vi "snapAndEnqueueTester.vi"(11 "Session In":T2) -> ()   [LabVIEW 2013]
uses:
  <vilib>/userdefined/High Color/IMAQdx.ctl
  <vilib>/vision/driver/NI_Vision_Acquisition_Software.lvlib
  <resource>/objmgr/imaqdx.rc
panel:
  in  "stop":bool
  out "Image":T1(plugin-control)
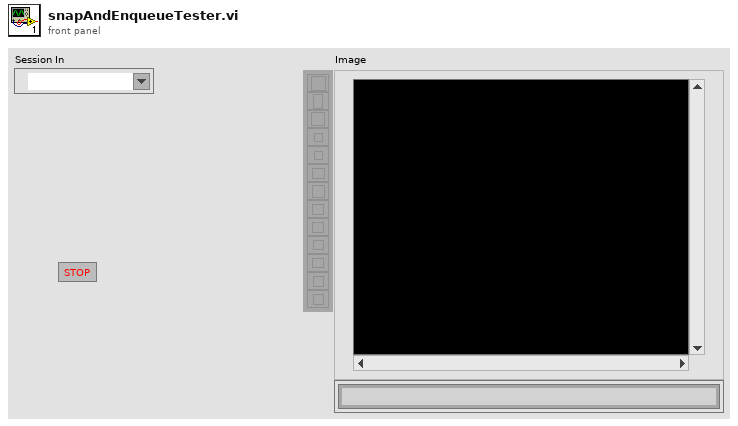
[diagram p1: front panel]
types:
  T1 = typedef "IMAQ Image.ctl" = refnum<image>
  T2 = typedef "IMAQdx.ctl" = refnum<k21>
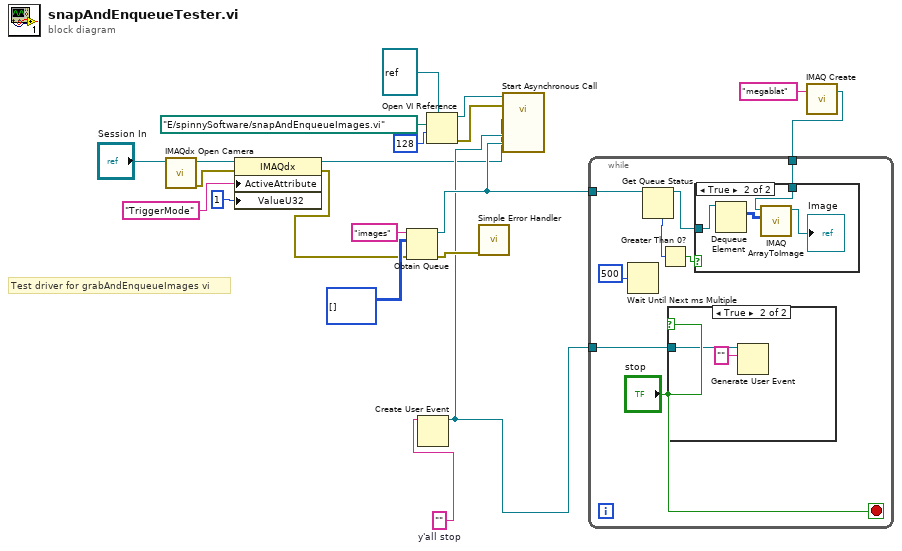
[diagram p0: block diagram]
diagram:
  w4 = ""  # y'all stop
  # "Test driver for grabAndEnqueueImages vi"
  n1 = call <vilib>:"IMAQdx Open Camera.vi"("Session In"="Session In") -> ("error out"=w16:errorcluster, "Session Out"=w19:T2)  [unwired: 9 in]
  n2 = property class="IMAQdx"(reference=w19, error in=w16, "ActiveAttribute"="TriggerMode", "ValueU32"=u32 1) -> (reference out=w2:T2, error out=w1:errorcluster)
  n3 = Obtain Queue(name (unnamed)="images", element data type=u8[][] [] ("Image Pixels (U8)"), error in (no error)=w1) -> (queue out=w7:refnum<queue>, error out=w15:errorcluster)  [unwired: 2 in, 1 out]
  n4 = Create User Event(user event datatype=w4) -> (user event=w3:refnum<user-event>)  [unwired: 1 in, 1 out]
  n5 = Open VI Reference(type specifier VI Refnum (for type only)=refnum<vi> refnum, vi path=path "E:/spinnySoftware/snapAndEnqueueImages.vi", options=128) -> (vi reference=w11:refnum<vi>, error out=w10:errorcluster)  [unwired: 3 in]
  n6 = call <vilib>:"Simple Error Handler.vi"("error in (no error)"=w15) -> ()  [unwired: 4 in, 5 out]
  n7 = call-by-ref "Start Asynchronous Call"(reference=w11, error in=w10, "queue in"=w7, "user event in"=w3, "Session In"=w2) -> ()  [unwired: 9 in, 2 out]
  n8 = call "IMAQ Create"("Image Name"="megablat") -> ("New Image"=w6:T1)  [unwired: 4 in, 1 out]
  n9 = while {
    tunnel: w7 -> [w24]
    tunnel: w6 -> [w23]
    tunnel: w3 -> [w22]
    stop <- "stop" stop-if-true
    n10 = Wait Until Next ms Multiple(millisecond multiple=u32 500) -> ()  [unwired: 1 out]
    n11 = Get Queue Status(queue=w24) -> (queue out=w28:refnum<queue>, # elements in queue=w25:i32)  [unwired: 2 in, 6 out]
    n12 = Greater Than 0?(x=w25) -> (x > 0?=w26:bool)
    n13 = case shown="True" "stop" {
      tunnel: w22 -> [_ w30]
      frame False {
      }
      frame True {
        n14 = Generate User Event(user event=w30, event data cluster="" ("event data")) -> ()  [unwired: 2 in, 2 out]
      }
    }
    n15 = case shown="True" w26 {
      tunnel: w28 -> [_ w34]
      tunnel: w23 -> [_ w31]
      frame False {
      }
      frame True {
        n16 = Dequeue Element(queue=w34) -> (element=w33:u8[][])  [unwired: 2 in, 3 out]
        n17 = call "IMAQ ArrayToImage"("Image Pixels (U8)"=w33, "Image"=w31) -> ("Image Out"=→"Image":T1)  [unwired: 8 in, 1 out]
      }
    }
  }
